vi "Demo.vi"() -> ()   [LabVIEW 2021, in "BluePlotDemo.lvlib"]
uses:
  Demo/BluePlotDemo.lvlib
  TypeDefs/plot load data V2.ctl
  TypeDefs/plot properties V2.ctl
  TypeDefs/plot attributes V2.ctl
  TypeDefs/Plot scale axis properties.ctl
  TypeDefs/Plot general properties.ctl
  Demo/SubVIs/ring buffer data.ctl
  Demo/Classes/BluePlotHandleDemo/BluePlotHandleDemo.lvclass
  C:/Code/open source/BluePlot/Source/Classes/BluePlotHandle/BluePlotHandle.lvclass
  Classes/BluePlotHandle/New Process.vi
  Classes/BluePlotHandle/Shutdown.vi
  Classes/BluePlotHandle/Get PlotConfig.vi
  Classes/BluePlotHandle/Load PlotConfig.vi
  <vilib>/National Instruments/Variant Ring Buffer/Ring Buffer.lvclass
  BluePlot.lvlib
  Classes/BluePlotHandle/BluePlotHandle.lvclass
  C:/Code/open source/BluePlot/Source/Demo/Classes/BluePlotHandleDemo/BluePlotHandleDemo.lvclass
panel:
  in  "load config":bool
  in  "get config":bool
  out "time to plot":dbl
  out "Subscribed names":i32(listbox)
  in  "Plot config":T1={"plots"=[], "X-axis"={"Name Label.Text"="", "Style"=0, "Tick Colors:Minor Tick Color"=0, "Tick Colors:Tick Color"=0, "Marker Colors:Text Color"=0, "Grid Colors:Major Color"=0, "Grid Colors:Minor Color"=0, "Mapping Mode"=0, "Flipped"=FALSE, "Name Label.Visible"=FALSE, "Name Label.Text Colors:Text Color"=0, "Scale Fit"=0, "Editable"=FALSE, "Range:Maximum"=0.0, "Range:Minimum"=0.0, "Offset and Multiplier:Multiplier"=0.0, "Offset and Multiplier:Offset"=0.0, "Name Label.Font:Size"=0, "Marker.Font:Size"=0, "Uniform Marker Spacing?"=TRUE, "Format String"=""}, "Y-axes"=[], "General"={"Title"="", "Time to Plot"=1800.0, "Title.Visible"=FALSE, "Legend:Visible"=FALSE, "Plot Area:Colors:BG Color"=0}} {"General"."Time to Plot" format="%<%M:%S>t"}
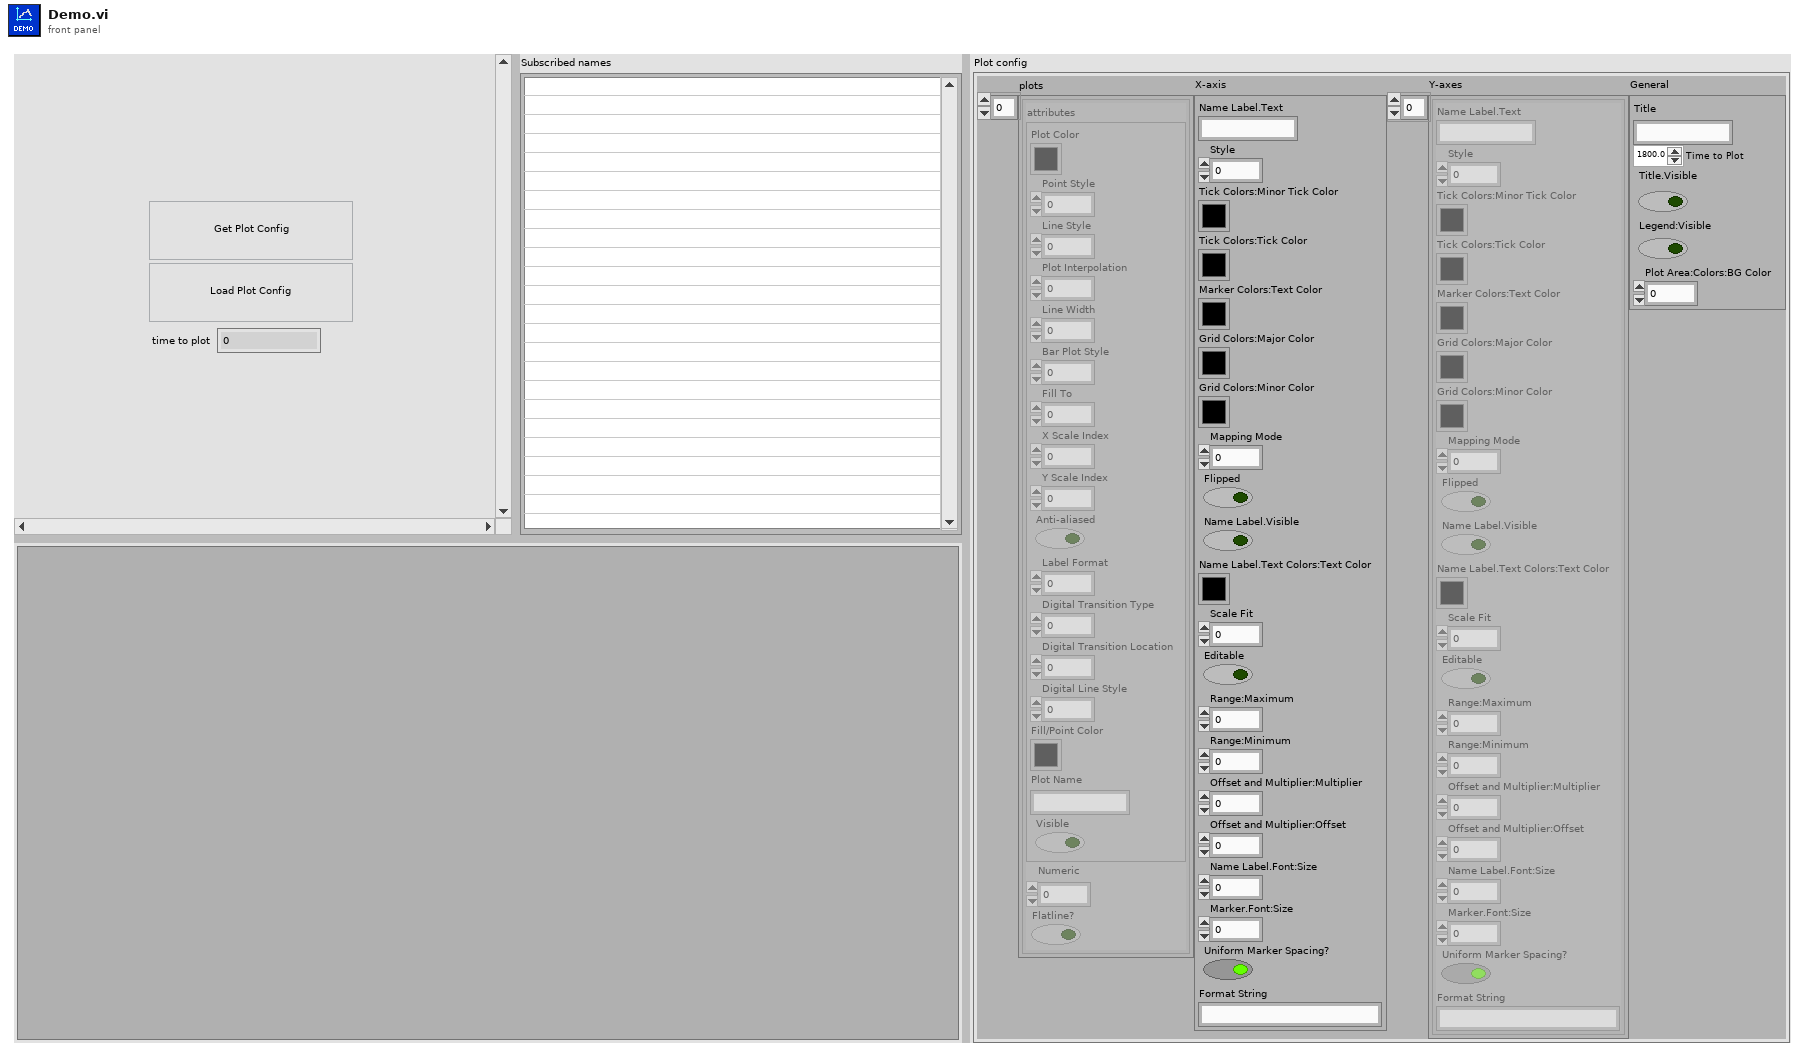
[diagram p1: front panel]
types:
  T1 = typedef "BluePlot.lvlib/plot load data V2.ctl" = cluster{"plots":T2[], "X-axis":T4, "Y-axes":T4[], "General":T5}
  T2 = typedef "BluePlot.lvlib/plot properties V2.ctl" = cluster{"attributes":T3, "Numeric":dbl, "Flatline?":bool}
  T3 = typedef "BluePlot.lvlib/plot attributes V2.ctl" = cluster{"Plot Color":u32, "Point Style":u8, "Line Style":u8, "Plot Interpolation":u8, "Line Width":u8, "Bar Plot Style":u8, "Fill To":i16, "X Scale Index":u32, "Y Scale Index":u32, "Anti-aliased":bool, "Label Format":u8, "Digital Transition Type":u8, "Digital Transition Location":u8, "Digital Line Style":u8, "Fill/Point Color":u32, "Plot Name":string, "Visible":bool}
  T4 = typedef "BluePlot.lvlib/Plot scale axis properties.ctl" = cluster{"Name Label.Text":string, "Style":u8, "Tick Colors:Minor Tick Color":u32, "Tick Colors:Tick Color":u32, "Marker Colors:Text Color":u32, "Grid Colors:Major Color":u32, "Grid Colors:Minor Color":u32, "Mapping Mode":u8, "Flipped":bool, "Name Label.Visible":bool, "Name Label.Text Colors:Text Color":u32, "Scale Fit":u8, "Editable":bool, "Range:Maximum":dbl, "Range:Minimum":dbl, "Offset and Multiplier:Multiplier":dbl, "Offset and Multiplier:Offset":dbl, "Name Label.Font:Size":u32, "Marker.Font:Size":u32, "Uniform Marker Spacing?":bool, "Format String":string}
  T5 = typedef "BluePlot.lvlib/Plot general properties.ctl" = cluster{"Title":string, "Time to Plot":dbl, "Title.Visible":bool, "Legend:Visible":bool, "Plot Area:Colors:BG Color":u32}
  T6 = typedef "BluePlotDemo.lvlib/Demo Names.ctl" = enum16{"Sine Wave", "Triangle Wave", "Sawtooth Wave", "Square Wave", "Uniform Noise", "Periodic Noise", "White Noise"}
  T7 = cluster{"subscribed names":refnum<user-event>, "time to plot":refnum<user-event>}
  T8 = typedef "BluePlotDemo.lvlib/ring buffer data.ctl" = cluster{"timestamp":dbl, "value":dbl}
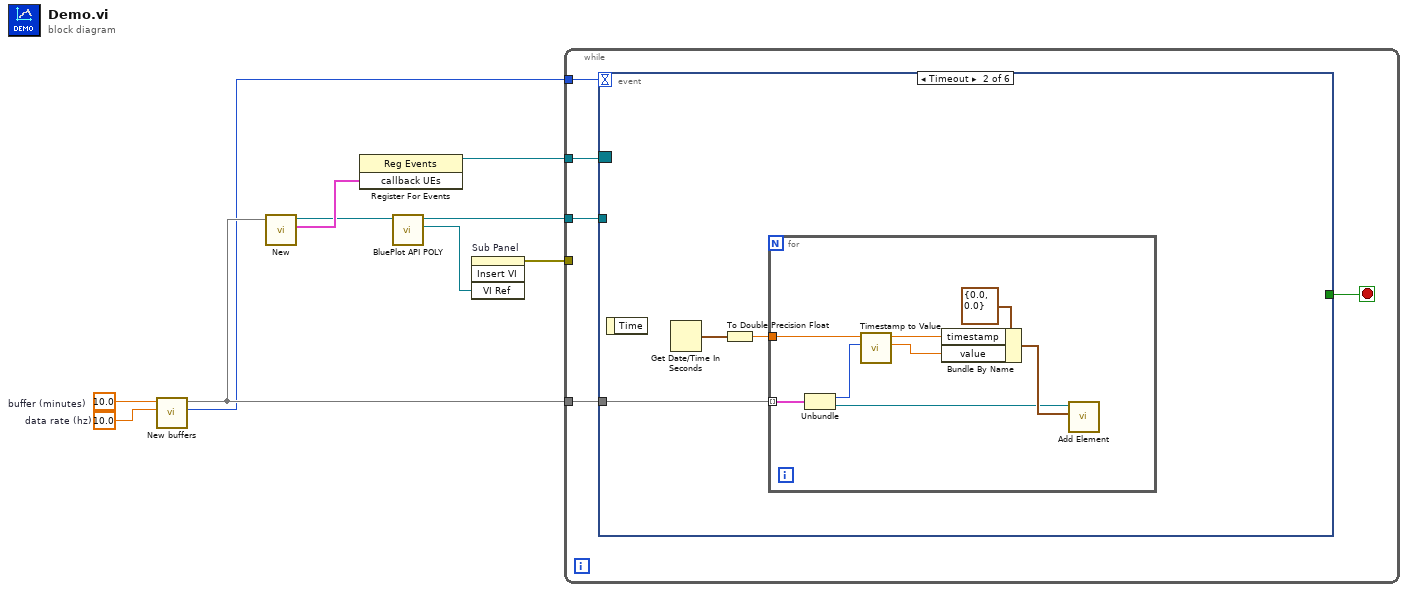
[diagram p0: block diagram]
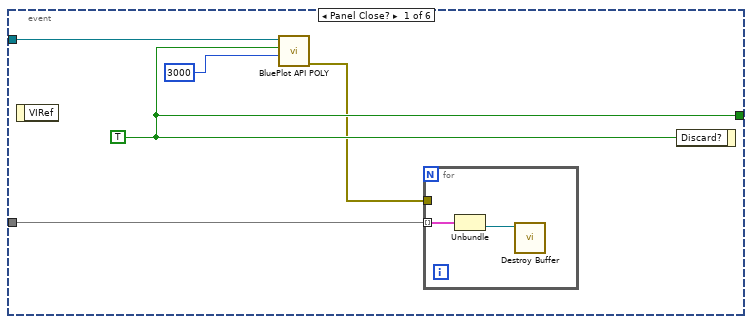
[diagram p2: hidden frame]
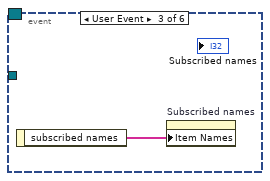
[diagram p3: hidden frame]
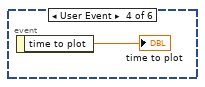
[diagram p4: hidden frame]
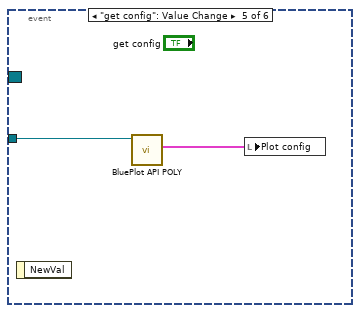
[diagram p5: hidden frame]
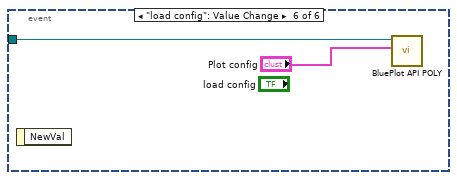
[diagram p6: hidden frame]
diagram:
  w7 = 10.0  # data rate (hz)
  w8 = 10.0  # buffer (minutes)
  n1 = call "New buffers.vi"("data rate (hz)"=w7, "buffer (minutes)"=w8) -> ("period (ms)"=w5:i32, "ChannelMap"=w6:map{T6, refnum<data-value>})  [unwired: 8 in]
  n2 = call "New.vi"("ChannelMap"=w6) -> ("callback UEs"=w10:T7, "BluePlotHandleDemo out"=w3:refnum<class "BluePlotHandleDemo.lvclass">)  [unwired: 8 in, 1 out]
  n3 = register-events(w10) -> (reference out=w9:refnum<event-registration>)  [unwired: 2 in, 1 out]
  n4 = call-poly "BluePlot API POLY.vi"("BluePlotHandle in"=w3) -> ("VI ref"=w1:refnum<vi>, "BluePlotHandle out"=w2:refnum<class "BluePlotHandleDemo.lvclass">)  [unwired: 8 in, 1 out]
  n5 = invoke on="Sub Panel" class="SubPnl" method="Insert VI"("VI Ref"=w1) -> (error out=w4:errorcluster)  [unwired: 3 in, 3 out]
  n6 = while {
    tunnel: w2 -> [w15]
    tunnel: w9 -> [w13]
    tunnel: w6 -> [w12]
    tunnel: w5 -> [w11]
    tunnel: w4 -> [_]
    stop <- w14 stop-if-true
    n7 = event shown="[1] Timeout" {
      selector: w13 -> [_ _ _ _ _ _]
      dyn-events: _ -> [_ _ _ _ _ _]
      timeout: w11 -> [_ _ _ _ _ _]
      tunnel: w15 -> [w19 _ _ _ w37 w39]
      tunnel: [w18 _ _ _ _ _] -> w14
      tunnel: w12 -> [w20 w25 _ _ _ _]
      event Panel Close? {
        w18 = TRUE ("Discard?")
        n8 = event-data() -> ()  [unwired: 1 in, 1 out]
        n9 = call-poly "BluePlot API POLY.vi"("wait timeout in ms (-1)"=3000, "Wait until shutdown? (F)"=w18, "BluePlotHandle in"=w19) -> ("error out"=w16:errorcluster)  [unwired: 8 in]
        n10 = for {
          tunnel: w16 -> [_]
          tunnel: w20 -> [w22] mode=indexing
          n11 = Unbundle(w22) -> ("Ring Buffer"=w21:refnum<data-value>)  [unwired: 1 out]
          n12 = call <vilib>:"Destroy Buffer.vi"("Ring Buffer Reference"=w21) -> ()  [unwired: 9 in, 2 out]
        }
        n13 = event-data("Discard?"=w18) -> ()  [unwired: 1 in, 1 out]
      }
      event Timeout {
        n14 = event-data() -> ()  [unwired: 1 in, 1 out]
        n15 = Get Date/Time In Seconds() -> (seconds since 1Jan1904=w24:timestamp)
        n16 = To Double Precision Float(number=w24) -> (double precision float=w23:dbl)
        n17 = for {
          tunnel: w25 -> [w28] mode=indexing
          tunnel: w23 -> [w33]
          n18 = Unbundle(w28) -> ("channel"=w27:T6, "Ring Buffer"=w26:refnum<data-value>)
          n19 = call "Timestamp to Value.vi"("Channel"=w27, "timestamp"=w33) -> ("value"=w30:dbl, "timestamp (dup)"=w31:dbl)  [unwired: 8 in]
          n20 = Bundle By Name(cluster=T8 {"timestamp"=0.0, "value"=0.0} ("Cluster"), "timestamp"=w31, "value"=w30) -> (w29:T8)
          n21 = call <vilib>:"Add Element.vi"("Variant"=w29, "Ring Buffer Reference"=w26) -> ()  [unwired: 8 in, 2 out]
        }
      }
      event User Event {
        n22 = event-data() -> ("subscribed names"=w34:string[])  [unwired: 1 in]
        n23 = property on="Subscribed names" class="LstBox (strict)"("Item Names"=w34) -> ()  [unwired: 2 in, 2 out]
      }
      event User Event {
        n24 = event-data() -> ("time to plot"=→"time to plot":dbl)  [unwired: 1 in]
      }
      event "get config": Value Change {
        n25 = event-data() -> ()  [unwired: 1 in, 1 out]
        n26 = call-poly "BluePlot API POLY.vi"("BluePlotHandle in"=w37) -> ("Plot config"=w36:T1)  [unwired: 8 in, 2 out]
        n27 = local write "Plot config"(w36) -> ()
      }
      event "load config": Value Change {
        n28 = event-data() -> ()  [unwired: 1 in, 1 out]
        n29 = call-poly "BluePlot API POLY.vi"("Plot config"="Plot config", "BluePlotHandle in"=w39) -> ()  [unwired: 8 in, 2 out]
      }
    }
  }
